vi "Read DI.vi"(0 "FPGA DI Loop Data in":T1={"DI"=[FALSE, FALSE, FALSE, FALSE, FALSE, FALSE, FALSE, FALSE, FALSE, FALSE, FALSE, FALSE, FALSE, FALSE, FALSE, FALSE, FALSE, FALSE, FALSE, FALSE, FALSE, FALSE, FALSE, FALSE, FALSE, FALSE, FALSE, FALSE, FALSE, FALSE, FALSE, FALSE], "Set Time uSec"=[0, 0, 0, 0, 0, 0, 0, 0, 0, 0, 0, 0, 0, 0, 0, 0, 0, 0, 0, 0, 0, 0, 0, 0, 0, 0, 0, 0, 0, 0, 0, 0]}, 1 "Cycles to Filter":u16=5) -> (4 "FPGA DI Loop Data out":T1, 6 "DI":u32, 15 "error out":errorcluster)   [LabVIEW 2019]
uses:
  TypeDef/FPGA DI Loop Data.ctl
  <vilib>/rvi/eio/common/nirviEmuTemplateMethod_errors.vi
  <vilib>/eio/EIONode/EIONode.xnode
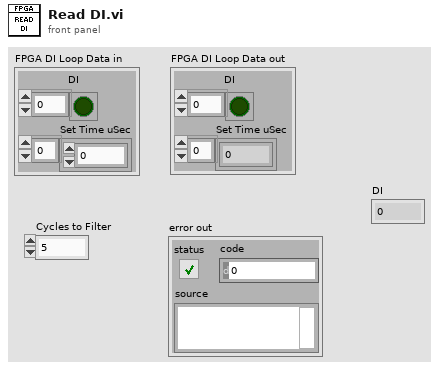
[diagram p1: front panel]
types:
  T1 = typedef "FPGA DI Loop Data.ctl" = cluster{"DI":bool[], "Set Time uSec":u16[]}
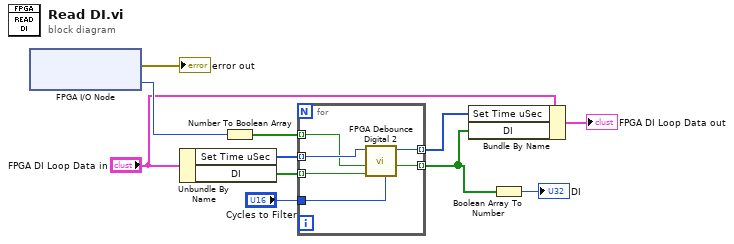
[diagram p0: block diagram]
diagram:
  n1 = xnode "FPGA I/O Node"() -> ("error out"=→"error out":errorcluster, "Mod1/DI31:0"=w11:u32)  [unwired: 2 in, 1 out]
  n2 = Unbundle By Name("FPGA DI Loop Data in") -> ("Set Time uSec"=w3:u16[], "DI"=w5:bool[])
  n3 = Number To Boolean Array(number=w11) -> (Boolean array=w7:bool[])
  n4 = for {
    tunnel: w3 -> [w16] mode=indexing
    tunnel: [w15] -> w2 mode=indexing
    tunnel: [w17] -> w6 mode=indexing
    tunnel: w7 -> [w14] mode=indexing
    tunnel: w5 -> [w13] mode=indexing
    tunnel: "Cycles to Filter" -> [w12]
    n5 = call "FPGA Debounce Digital 2.vi"("Cycles to Filter"=w12, "Previous Output Signal"=w13, "Input Signal"=w14, "tick in"=w16) -> ("Output Filtered Signal"=w15:bool, "tick out"=w17:u16)  [unwired: 6 in]
  }
  n6 = Bundle By Name(cluster="FPGA DI Loop Data in", "Set Time uSec"=w6, "DI"=w2) -> (→"FPGA DI Loop Data out":T1)
  n7 = Boolean Array To Number(Boolean array=w2) -> (number=→"DI":u32)
